vi "handshakeSimulTest.vi"() -> ()   [LabVIEW 2014]
uses:
  <vilib>/Platform/TimedLoop/XDataNode/timing_clust.ctl
  <vilib>/Platform/TimedLoop/XDataNode/nitl_modes.ctl
  <vilib>/Platform/TimedLoop/XDataNode/wakeup.ctl
  <vilib>/rvi/Emulation/niFpgaGetClockAttributes.vi
  <vilib>/rvi/Emulation/niFpgaSctlEmulationGetInTimedLoop.vi
  <vilib>/rvi/Emulation/niFpgaEmulationReportErrorSimple.vi
  <vilib>/rvi/Emulation/niFpgaCriticalErrorInLSC.vi
  <vilib>/rvi/Emulation/niFpgaEmulationIsFPGAContextNoSignature.vi
  <vilib>/rvi/DataTransferAndStorage/Container/Common/niFpgaContainerGetUniqueNameForEmu.vi
  <vilib>/rvi/eio/common/nirviEmuReportErrorAndStop.vi
  <vilib>/rvi/Emulation/niFpgaProcessEmulError.vi
  <vilib>/rvi/eio/common/nirviEmuTemplateMethod_errors.vi
  <vilib>/Platform/TimedLoop/XDataNode/XDataNode.xnode
  <vilib>/rvi/DataTransferAndStorage/Container/XNode/niFpgaContainer.xnode
  <vilib>/rvi/DataTransferAndStorage/Handshake/Emulation/niFpgaHandshakeEmulation.vi
  <vilib>/eio/EIONode/EIONode.xnode
  <vilib>/Platform/TimedLoop/XDataNode/XDNodeRunTimeDep.lvlib
panel:
  in  "stop 2":bool
  out "Numeric":i32
  in  "stop":bool
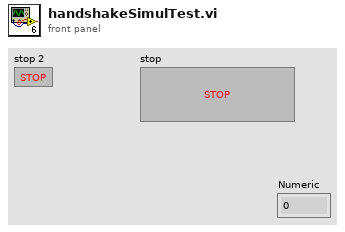
[diagram p1: front panel]
types:
  T1 = typedef "XDNodeRunTimeDep.lvlib/timing_clust.ctl" = cluster{"Expected End [f-1]":u64, "Actual End [f-1]":u64, "Finished Late? [f-1]":bool, "Expected End [i-1]":u64, "Actual End [i-1]":u64, "Finished Late? [i-1]":bool, "Expected Start [i]":u64, "Actual Start [i]":u64, "Expected Start [f]":u64, "Actual Start [f]":u64, "Source Name":string, "Structure Name":string, "Period":i64, "Deadline":i64, "Offset":i64, "Start":i64, "Priority":i32, "Timeout":i32, "Mode":T2, "Wakeup Reason":T3, "Error":errorcluster, "Source Type":string, "Secondary Source Type":string, "Global End Time":u64, "Global Start Time":u64, "Frame Duration":u64, "Iteration Duration":u64, "Assigned CPU":i32, "I/O Scan Engine Mode":u32}
  T2 = typedef "XDNodeRunTimeDep.lvlib/nitl_modes.ctl" = enum32{"No Change", "Process missed periods, maintain original phase", "Discard missed periods, maintain original phase", "Process missed periods, ignore original phase", "Discard missed periods, ignore original phase"}
  T3 = typedef "XDNodeRunTimeDep.lvlib/wakeup.ctl" = enum32{"Normal", "Aborted", "Asynchronous wakeup", "Timing source error", "Timed loop error", "Timeout"}
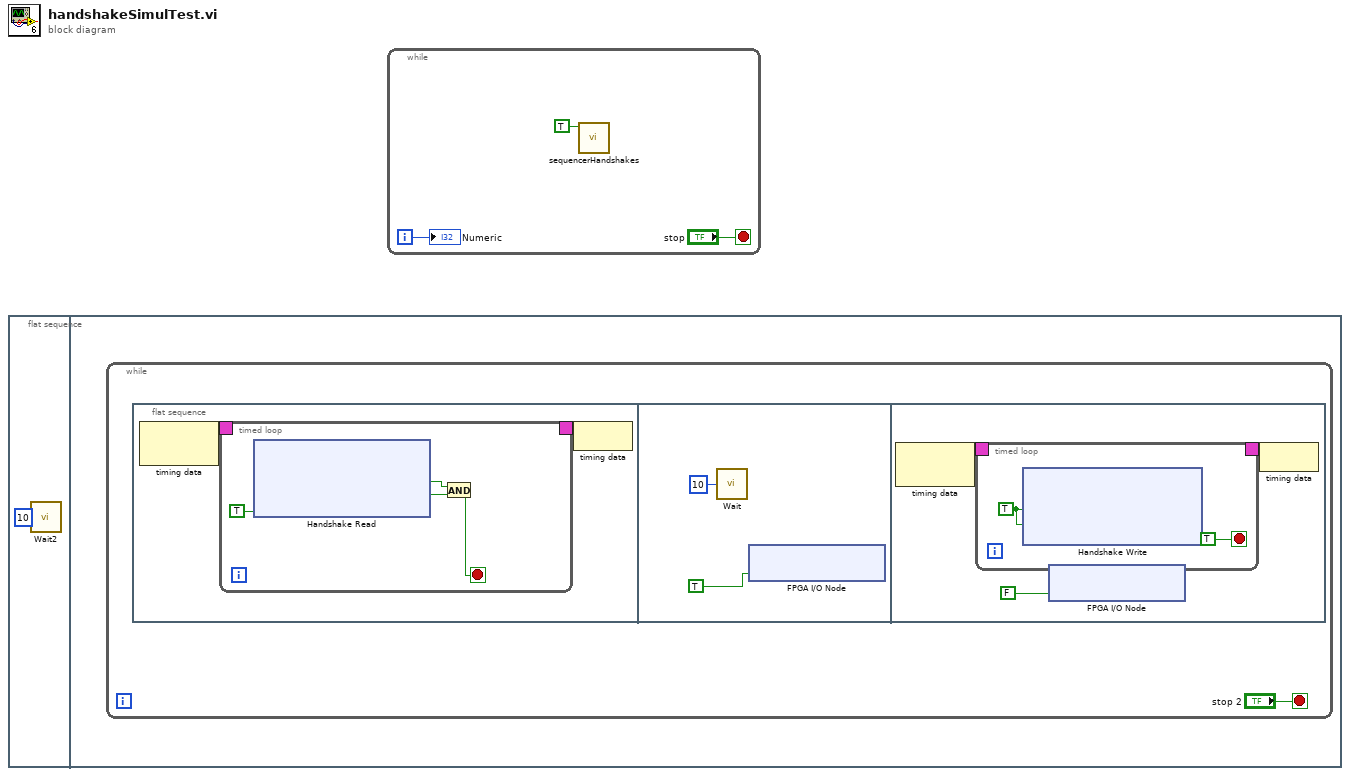
[diagram p0: block diagram]
diagram:
  n1 = flat-sequence {
    frame #0 {
      n2 = call "Wait2"("Count(mSec)"=u32 10) -> ()  [unwired: 1 out]
    }
    frame #1 {
      n3 = while {
        stop <- "stop 2" stop-if-true
        n4 = flat-sequence {
          frame #0 {
            n5 = node-c288() -> (w4:T1)  [unwired: 1 in]
            n6 = timed-loop {
              timing: w4 -> [_]
              timing-out: [_] -> w3
              stop <- w6 stop-if-true
              n7 = xnode "Handshake Read"("Ready for Output"=TRUE) -> ("Data"=w8:bool, "Output Valid"=w7:bool)  [unwired: 1 in, 1 out]
              n8 = And(x=w8, y=w7) -> (x .and. y?=w6:bool)
            }
            n9 = node-c288(w3) -> ()
          }
          frame #1 {
            n10 = call "Wait"("Count(Ticks)"=u32 10) -> ()  [unwired: 1 out]
            n11 = xnode "FPGA I/O Node"("Connector1/DIO3"=TRUE ("handshookWait")) -> ()  [unwired: 1 in, 1 out]
          }
          frame #2 {
            n12 = node-c288() -> (w17:T1)  [unwired: 1 in]
            n13 = timed-loop {
              timing: w17 -> [_]
              timing-out: [_] -> w16
              stop <- TRUE stop-if-true
              w19 = TRUE ("Data")
              n14 = xnode "Handshake Write"("Data"=w19, "Input Valid"=w19) -> ()  [unwired: 1 in, 2 out]
            }
            n15 = xnode "FPGA I/O Node"("Connector1/DIO3"=FALSE ("handshookWait")) -> ()  [unwired: 1 in, 1 out]
            n16 = node-c288(w16) -> ()
          }
        }
      }
    }
  }
  n17 = while {
    i -> [w24]
    stop <- "stop" stop-if-true
    n18 = call "sequencerHandshakes.vi"("kepcoScan/MCS"=TRUE) -> ()  [unwired: 11 in]
    "Numeric" <- w24
  }
